vi "Init Trigger.vi"(8 "error in":errorcluster, 11 "VISA resource name in":refnum<visa-resource-name>) -> (0 "error out":errorcluster, 3 "VISA resource name out":refnum<visa-resource-name>)   [LabVIEW 2021, in "Keysight U1282A.lvlib"]
doc: "El comando INIT saca al instrumento U1282A del estado de espera y manda un redisparo cuando el instrumento está en modo trigger hold."
uses:
  Keysight U1282A.lvlib
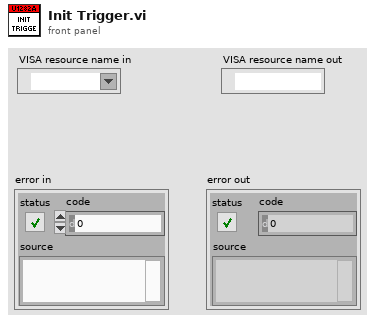
[diagram p1: front panel]
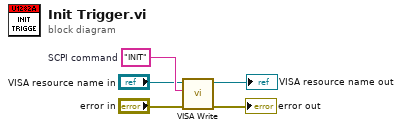
[diagram p0: block diagram]
diagram:
  w5 = "INIT"  # SCPI command
  n1 = call "VISA Write.vi"("error in"="error in", "SCPI command"=w5, "VISA resource in"="VISA resource name in") -> ("error out"=→"error out":errorcluster, "VISA resource out"=→"VISA resource name out":refnum<visa-resource-name>)  [unwired: 6 in, 1 out]
